vi "Padding.vi"(9 "size":i32=8, 11 "bytes in":i32) -> (1 "padding":i32, 3 "total bytes":i32)   [LabVIEW 2022 SP3]
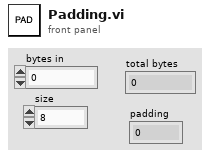
[diagram p1: front panel]
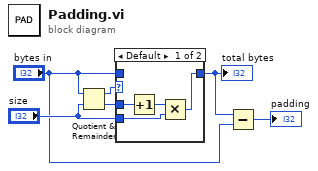
[diagram p0: block diagram]
diagram:
  n1 = Quotient & Remainder(x="bytes in", y="size") -> (x-y*floor(x/y)=w4:i32, floor(x/y)=w5:i32)
  n2 = case shown="Default" w4 {
    tunnel: [w7 w11] -> w3
    tunnel: "bytes in" -> [_ w11]
    tunnel: w5 -> [w10 _]
    tunnel: "size" -> [w8 _]
    frame Default {
      n3 = Increment(x=w10) -> (x+1=w9:i32)
      n4 = Multiply(x=w9, y=w8) -> (x*y=w7:i32)
    }
    frame 0 {
    }
  }
  "total bytes" <- w3
  n5 = Subtract(x=w3, y="bytes in") -> (x-y=→"padding":i32)
